vi "MD5 pad.vi"(9 "Message String Length (bytes)":i32, 10 "Last Part of Message String":string) -> (2 "Padding":string)   [LabVIEW 2016]
doc: "This VI creates a new string that represents the padding for the message string. The sum of the lengths of the message string and the padding string (in bytes) must be a multiple of 64."
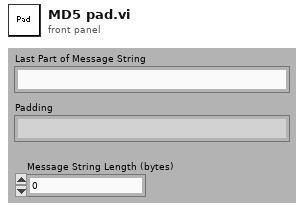
[diagram p1: front panel]
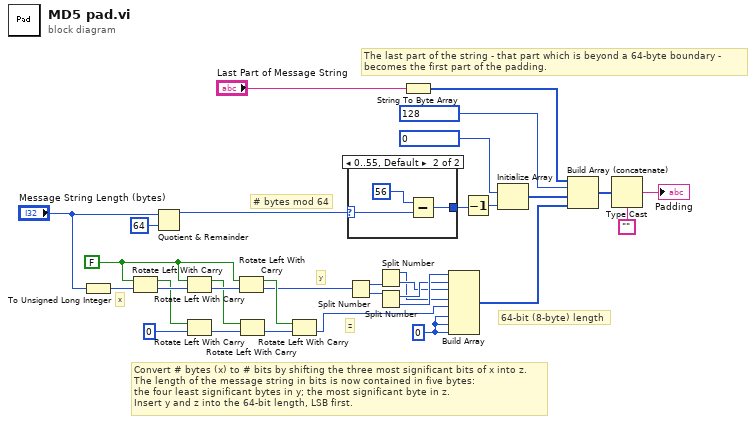
[diagram p0: block diagram]
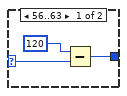
[diagram p2: hidden frame]
diagram:
  w18 = FALSE ("carry")
  w21 = u8 0
  # "The last part of the string - that part which is beyond a 64-byte boundary -\nbecomes the first part of the padding."
  # "64-bit (8-byte) length"
  # "x"
  # "y"
  # "z"
  # "Convert # bytes (x) to # bits by shifting the three most significant bits of x into z.\nThe length of the message string in bits is now contained in five bytes:  \nthe four least significant bytes in y; the most significant byte in z.\nInsert y and z into the 64-bit length, LSB first."
  # "# bytes mod 64"
  n1 = To Unsigned Long Integer(number="Message String Length (bytes)") -> (unsigned 32bit integer=w6:u32)
  n2 = Rotate Left With Carry(2:w6, 3:w18) -> (0:w19:u32, 1:w15:bool)
  n3 = Quotient & Remainder(x="Message String Length (bytes)", y=64) -> (x-y*floor(x/y)=w5:i32)  [unwired: 1 out]
  n4 = Rotate Left With Carry(2:w19, 3:w18) -> (0:w17:u32, 1:w13:bool)
  n5 = Rotate Left With Carry(2:u8 0, 3:w15) -> (0:w14:u8)  [unwired: 1 out]
  n6 = Rotate Left With Carry(2:w17, 3:w18) -> (0:w10:u32, 1:w11:bool)
  n7 = Rotate Left With Carry(2:w14, 3:w13) -> (0:w12:u8)  [unwired: 1 out]
  n8 = Rotate Left With Carry(2:w12, 3:w11) -> (0:w9:u8)  [unwired: 1 out]
  n9 = Split Number(x=w10) -> (hi(x)=w29:u16, lo(x)=w28:u16)
  n10 = case shown="0..55, Default" w5 {
    selector: w5 -> [w35 w38]
    tunnel: [w34 w37] -> w8
    frame 56..63 {
      n11 = Subtract(x=120, y=w35) -> (x-y=w34:i32)
    }
    frame 0..55, Default {
      n12 = Subtract(x=56, y=w38) -> (x-y=w37:i32)
    }
  }
  n13 = Split Number(x=w29) -> (hi(x)=w24:u8, lo(x)=w25:u8)
  n14 = Split Number(x=w28) -> (hi(x)=w26:u8, lo(x)=w27:u8)
  n15 = String To Byte Array(string="Last Part of Message String") -> (unsigned byte array=w7:u8[])
  n16 = Build Array(w27, w26, w25, w24, w9, w21, w21, w21) -> (w23:u8[])
  n17 = Decrement(x=w8) -> (x-1=w20:i32)
  n18 = Initialize Array(u8 0, w20) -> (w32:u8[])
  n19 = Build Array (concatenate)(w7, u8 128, w32, w23) -> (w22:u8[])
  n20 = Type Cast(type="", x=w22) -> (*(type *) &x=→"Padding":string)
